vi "PSAE_VCH_TempVariable.vi"() -> (1 "TempVariable":T2={"Error"={"status"=FALSE, "code"=0, "source"=""}, "Exit"=FALSE, "Local VIRef"=refnum, "Q_Local"={"Name"="", "Order"="", "Data"=variant}, "Q_High"={"Name"="", "Order"="", "Data"=variant}, "Q_Send"={"Name[]"=[], "Order[]"=[], "Data[]"=[]}, "Popup Index"=0, "Ref"={"VCHList"=refnum, "Message"=refnum}, "Q_VCHEG"="", "DAQ2ANA"=[{"Card Name"="9: NI PXIe-4300 \"PXI1Slot9\"", "Channels Tag"=["PXI1Slot9/ai0", "PXI1Slot9/ai1", "PXI1Slot9/ai2", "PXI1Slot9/ai3", "PXI1Slot9/ai4", "PXI1Slot9/ai5", "PXI1Slot9/ai6", "PXI1Slot9/ai7"], "Channels Name"=["", "", "", "", "", "", "", ""], "Unit"=[]}], "PopUp Name"="", "Symbol Path"=path ""})   [LabVIEW 2016]
uses:
  VCH/Private/Ctrls/PSVCH_All Channels.ctl
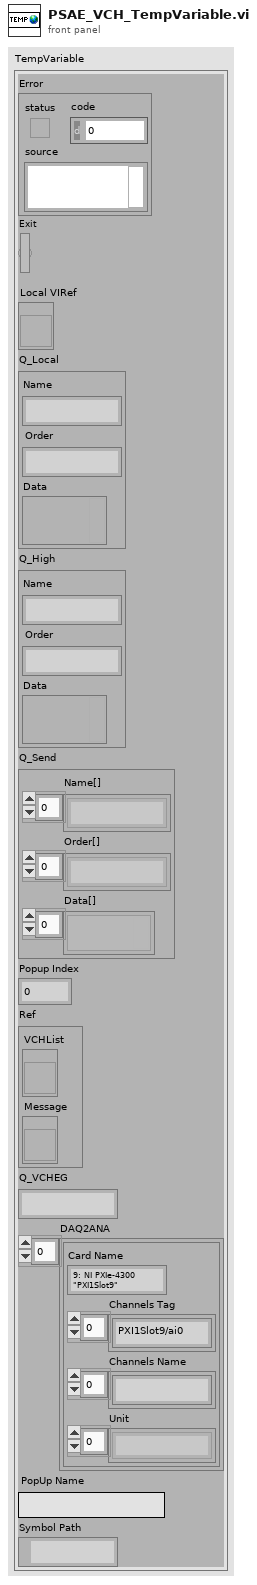
[diagram p1: front panel]
types:
  T1 = typedef "PSVCH_All Channels.ctl" = cluster{"Card Name":string, "Channels Tag":string[], "Channels Name":string[], "Unit":string[]}
  T2 = cluster{"Error":errorcluster, "Exit":bool, "Local VIRef":refnum<vi>, "Q_Local":cluster{"Name":string, "Order":string, "Data":variant}, "Q_High":cluster{"Name":string, "Order":string, "Data":variant}, "Q_Send":cluster{"Name[]":string[], "Order[]":string[], "Data[]":variant[]}, "Popup Index":i32, "Ref":cluster{"VCHList":refnum<vi>, "Message":refnum<vi>}, "Q_VCHEG":string, "DAQ2ANA":T1[], "PopUp Name":string, "Symbol Path":path}
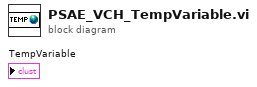
[diagram p0: block diagram]
diagram:
